vi "TCPSYN.vi"(5 "vi reference":refnum<vi>, 6 "Front Panel Window:Open":bool, 7 "error in vi ref":errorcluster, 8 "error in TCP":errorcluster, 9 "input Controls":cluster{"name":string, "type desc":i16[]}[](array[cluster]), 10 "input Indicators":cluster{"name":string, "type desc":i16[]}[](array[cluster]), 11 "connection ID in":refnum<k5>) -> (0 "error TCP out":errorcluster, 1 "error out":errorcluster, 2 "vi reference":refnum<vi>, 3 "connection ID out":refnum<k5>)   [LabVIEW 2010]
panel:
  out "error out 2":errorcluster
types:
  T1 = enum32{"Bad", "Idle", "Run top level", "Running"}
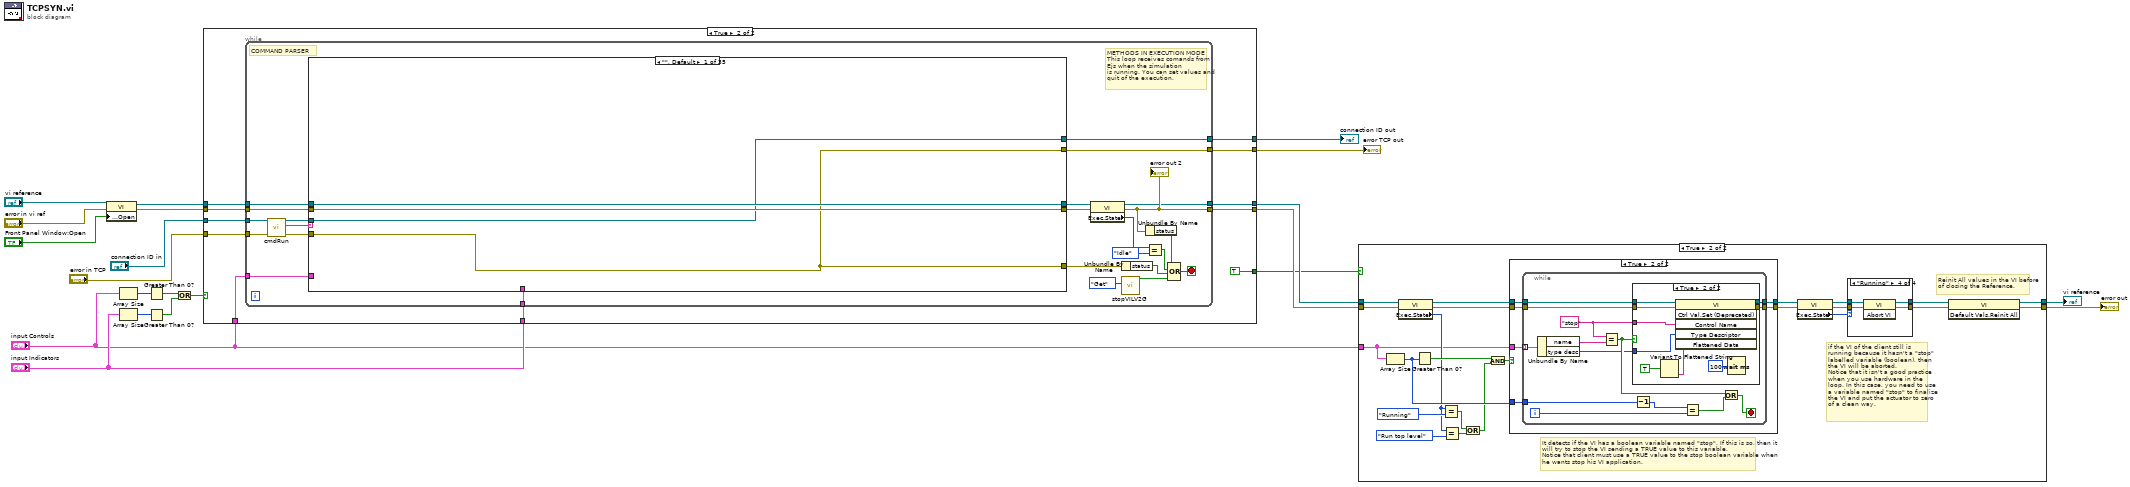
[diagram p0: block diagram]
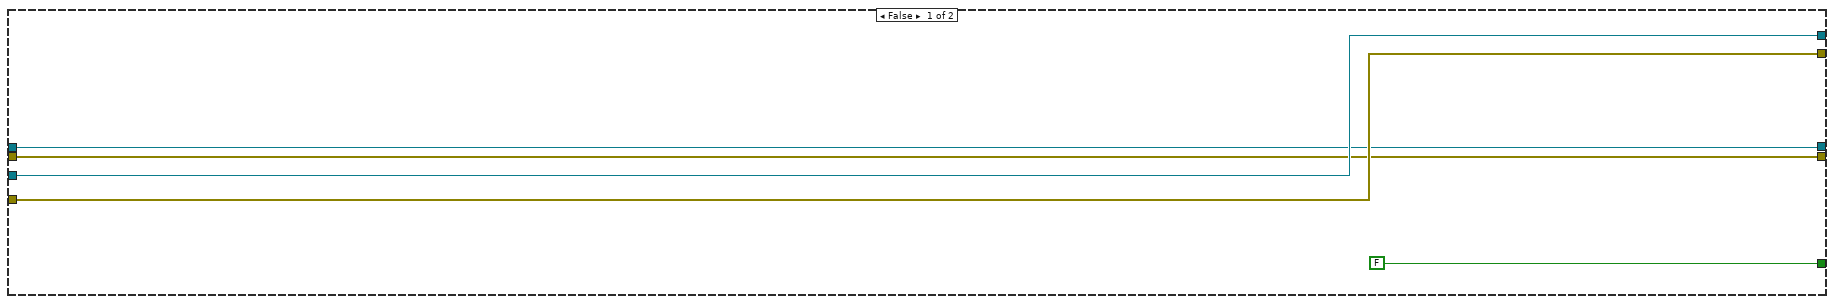
[diagram p8: hidden frame]
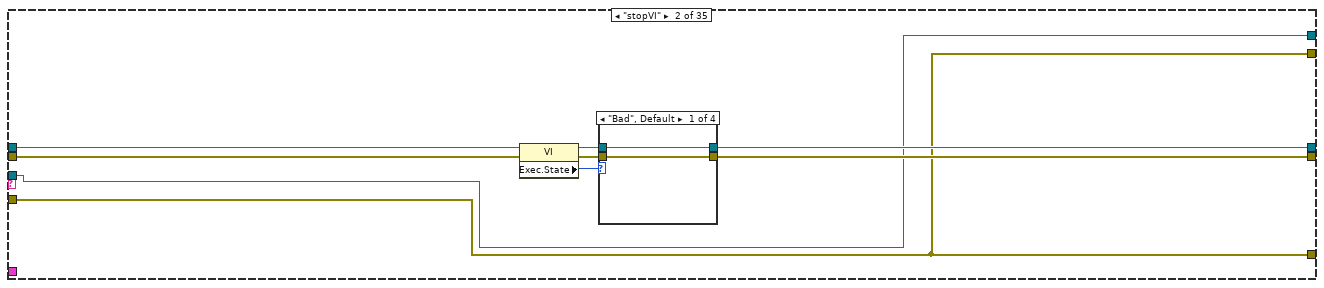
[diagram p9: hidden frame]
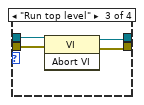
[diagram p11: hidden frame]
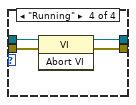
[diagram p12: hidden frame]
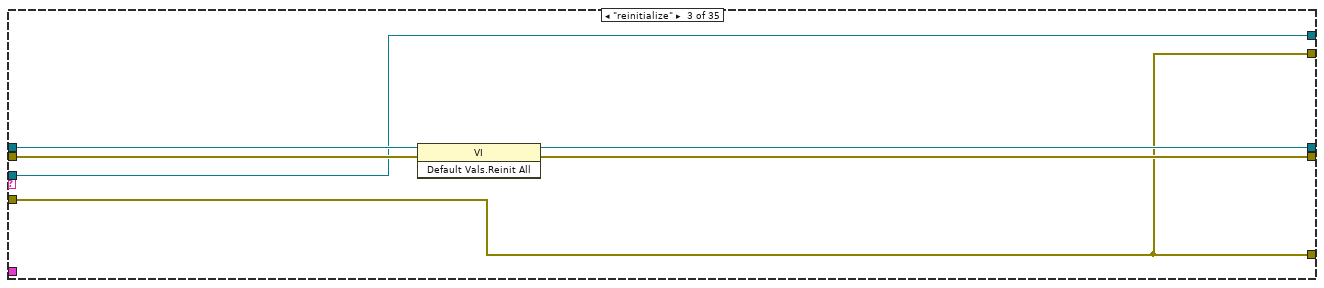
[diagram p13: hidden frame]
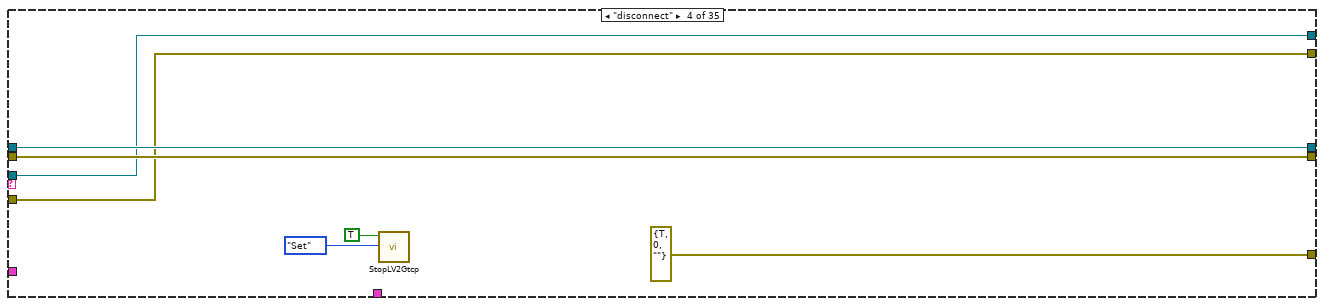
[diagram p14: hidden frame]
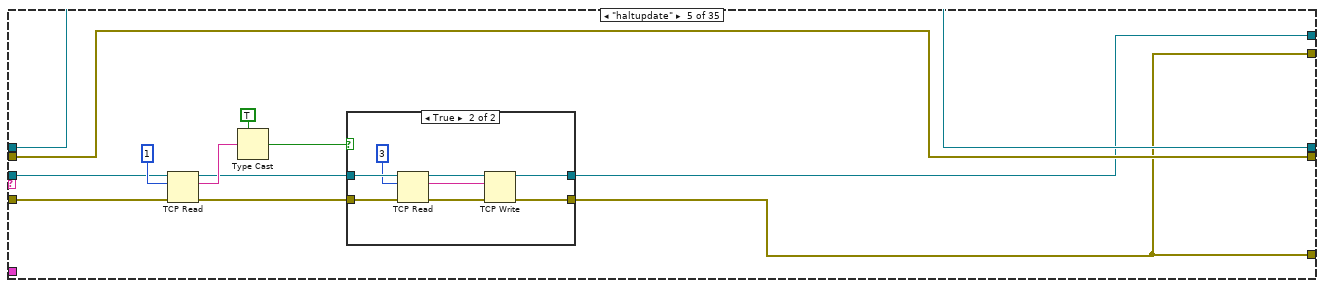
[diagram p15: hidden frame]
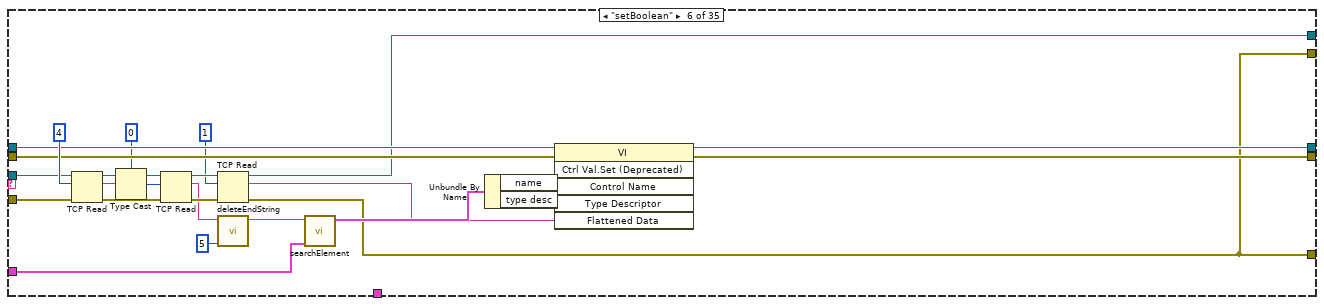
[diagram p17: hidden frame]
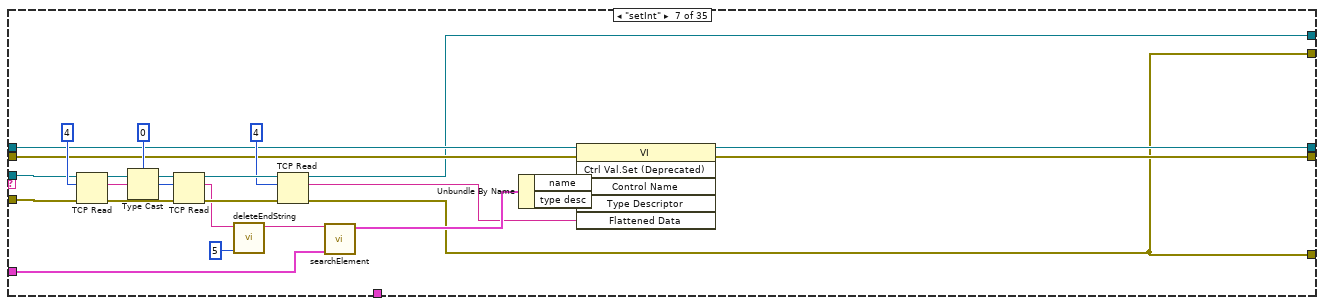
[diagram p18: hidden frame]
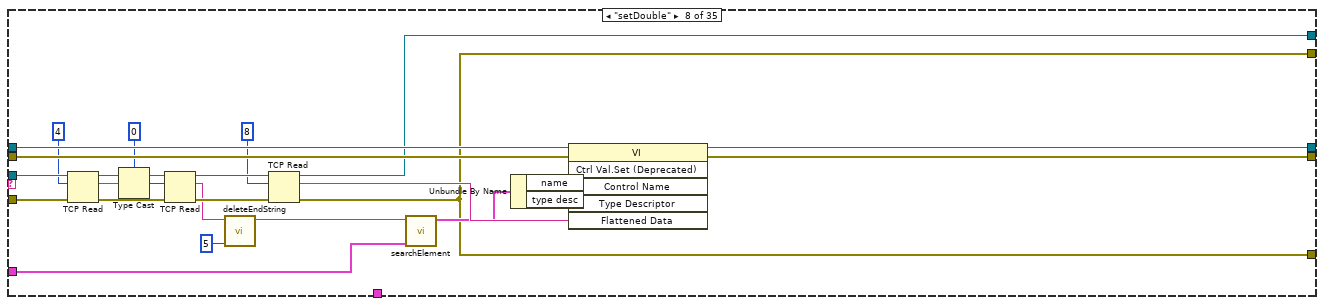
[diagram p19: hidden frame]
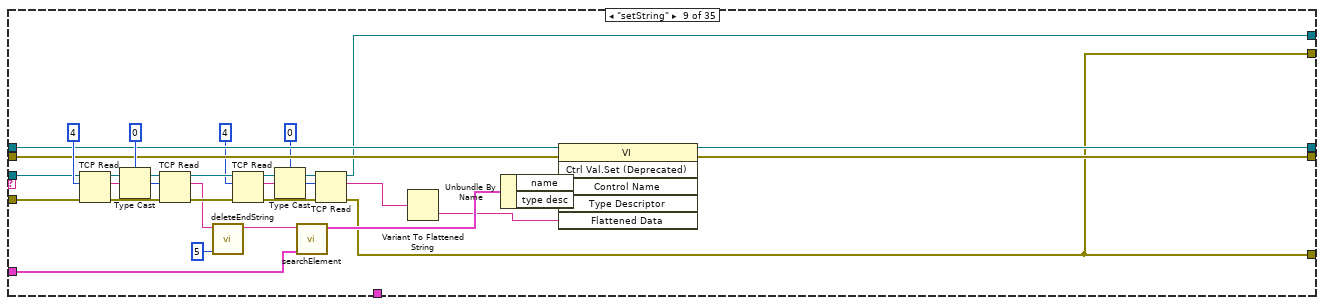
[diagram p20: hidden frame]
diagram:
  n1 = property on="Property Node" class="VI"(reference="vi reference", error in="error in vi ref", "Front Panel.Open"="Front Panel Window:Open") -> (reference out=w15:refnum<vi>, error out=w16:errorcluster)
  n2 = Array Size(array="input Controls") -> (size(s)=w14:i32)
  n3 = Array Size(array="input Indicators") -> (size(s)=w12:i32)
  n4 = Greater Than 0?(x=w14) -> (x > 0?=w13:bool)
  n5 = Greater Than 0?(x=w12) -> (x > 0?=w11:bool)
  n6 = Or(x=w13, y=w11) -> (x .or. y?=w9:bool)
  n7 = case shown="True" w9 {
    tunnel: "connection ID in" -> [w25 w37]
    tunnel: "error in TCP" -> [w24 w36]
    tunnel: "input Controls" -> [_ w35]
    tunnel: "input Indicators" -> [_ w34]
    tunnel: w15 -> [w23 w33]
    tunnel: w16 -> [w22 w32]
    tunnel: [FALSE TRUE] -> w2
    tunnel: [w22 w30] -> w4
    tunnel: [w23 w29] -> w3
    tunnel: [w25 w28] -> w8
    tunnel: [w24 w27] -> w7
    frame False {
    }
    frame True {
      n8 = while {
        tunnel: w37 -> [w58]
        tunnel: w36 -> [w57]
        tunnel: w33 -> [w61]
        tunnel: w32 -> [w60]
        tunnel: w35 -> [w52]
        tunnel: w34 -> [w43]
        tunnel: [w41] -> w30
        tunnel: [w40] -> w29
        tunnel: [w39] -> w28
        tunnel: [w38] -> w27
        stop <- w42 stop-if-true
        # "METHODS IN EXECUTION MODE\nThis loop receives comands from Ejs when the simulation\nis running. You can set values and quit of the execution."
        # "COMMAND PARSER"
        n9 = call "cmdRun.vi"("error in (no error)"=w57, "connection ID"=w58) -> ("error out"=w54:errorcluster, "Command"=w56:string, "connection ID out"=w55:refnum<k5>)  [unwired: 7 out]
        n10 = case shown="\"\", Default" w56 {
          tunnel: w61 -> [w64 w71 w92 w96 w103 w142 w152 w196 w216 w236 w256 w292 w341 _ w409 w441 w482 w530 w564 w620 w657 w684 w707 w725 w753 w773 w796 w819 w842 w867 w888 w911 w934 w957 w978]
          tunnel: w60 -> [w65 w70 w91 w95 w102 w141 w149 w195 w215 w235 w255 w291 w340 _ w408 w440 w481 w531 w563 w619 w656 w683 w706 w726 w752 w772 w797 w820 w843 w868 w889 w912 w935 w958 w977]
          tunnel: [w65 w68 w89 w95 w102 w139 w151 w194 w211 w232 w259 w293 w339 w363 w403 w442 w484 w528 w565 w615 w658 w681 w704 w728 w747 w770 w795 w818 w841 w862 w887 w910 w933 w956 w980] -> w48
          tunnel: w55 -> [w63 w67 w87 w93 w104 w138 w159 w192 w214 w231 w262 w296 w349 w367 w406 w445 w487 w545 w568 w618 w661 w679 w703 w730 w751 w774 w799 w821 w845 w866 w890 w914 w936 w959 w983]
          tunnel: w54 -> [w62 w66 w88 w94 w105 w137 w160 w193 w213 w230 w261 w295 w348 w366 w407 w444 w486 w544 w567 w617 w660 w678 w702 w729 w750 w775 w798 w822 w844 w865 w891 w913 w937 w960 w982]
          tunnel: [w62 w66 w88 errorcluster {"status"=TRUE, "code"=0, "source"=""} ("error out") w100 w123 w147 w172 w197 w228 w254 w290 w326 w361 w402 w437 w478 w519 w560 w612 w653 w676 w699 w722 w745 w768 w791 w814 w837 w860 w883 w906 w929 w952 w975] -> w53
          tunnel: w52 -> [_ _ _ _ _ w140 w154 w182 w212 w234 w258 w297 w344 w365 w405 w439 w483 w543 w562 w614 _ _ _ _ _ _ _ _ _ _ _ _ _ _ _]
          tunnel: [w64 w69 w90 w96 w103 w124 w150 w174 w199 w233 w260 w294 w327 w364 w404 w443 w485 w521 w566 w616 w659 w682 w705 w727 w748 w771 w794 w817 w840 w863 w886 w909 w932 w955 w979] -> w49
          tunnel: w43 -> [_ _ _ _ _ _ _ _ _ _ _ _ _ _ _ _ _ _ _ _ w655 w680 w701 w724 w749 w776 w793 w816 w839 w864 w885 w908 w931 w954 w981]
          tunnel: [w63 w67 w87 w93 w101 w122 w148 w173 w198 w229 w253 w289 w325 w362 w401 w438 w479 w520 w561 w613 w654 w677 w700 w723 w746 w769 w792 w815 w838 w861 w884 w907 w930 w953 w976] -> w39
          tunnel: [w62 w66 w88 w94 w100 w123 w147 w172 w197 w228 w254 w290 w326 w361 w402 w437 w478 w519 w560 w612 w653 w676 w699 w722 w745 w768 w791 w814 w837 w860 w883 w906 w929 w952 w975] -> w38
          frame "", Default {
          }
          frame "stopVI" {
            n11 = property class="VI"(reference=w71, error in=w70) -> (reference out=w73:refnum<vi>, error out=w72:errorcluster, "Exec.State"=w74:T1)
            n12 = case shown="\"Bad\", Default" w74 {
              tunnel: w73 -> [w76 w78 w82 w86]
              tunnel: w72 -> [w75 w77 w81 w85]
              tunnel: [w76 w78 w80 w84] -> w69
              tunnel: [w75 w77 w79 w83] -> w68
              frame "Bad", Default {
              }
              frame "Idle" {
              }
              frame "Run top level" {
                n13 = invoke class="VI" method="Abort VI"(reference=w82, error in=w81) -> (reference out=w80:refnum<vi>, error out=w79:errorcluster)  [unwired: 1 in, 1 out]
              }
              frame "Running" {
                n14 = invoke class="VI" method="Abort VI"(reference=w86, error in=w85) -> (reference out=w84:refnum<vi>, error out=w83:errorcluster)  [unwired: 1 in, 1 out]
              }
            }
          }
          frame "reinitialize" {
            n15 = invoke class="VI" method="Default Vals.Reinit All"(reference=w92, error in=w91) -> (reference out=w90:refnum<vi>, error out=w89:errorcluster)  [unwired: 1 in, 1 out]
          }
          frame "disconnect" {
            n16 = call "StopLV2Gtcp.vi"("Mode"=enum16{"Init", "Get", "Set"}."Set", "Stop IN"=TRUE) -> ()  [unwired: 10 out]
          }
          frame "haltupdate" {
            n17 = TCP Read(connection ID=w104, bytes to read=1, error in (no error)=w105) -> (connection ID out=w107:refnum<k5>, data out=w110:string, error out=w106:errorcluster)  [unwired: 2 out]
            n18 = Type Cast(type=TRUE, x=w110) -> (*(type *) &x=w108:bool)
            n19 = case shown="True" w108 {
              tunnel: w107 -> [w112 w121]
              tunnel: w106 -> [w113 w120]
              tunnel: [w113 w115] -> w100
              tunnel: [w112 w114] -> w101
              frame False {
              }
              frame True {
                n20 = TCP Read(connection ID=w121, bytes to read=3, error in (no error)=w120) -> (connection ID out=w119:refnum<k5>, data out=w117:string, error out=w118:errorcluster)  [unwired: 2 out]
                n21 = TCP Write(connection ID=w119, data in=w117, error in (no error)=w118) -> (connection ID out=w114:refnum<k5>, error out=w115:errorcluster)  [unwired: 2 out]
              }
            }
          }
          frame "setBoolean" {
            n22 = TCP Read(connection ID=w138, bytes to read=4, error in (no error)=w137) -> (connection ID out=w133:refnum<k5>, data out=w136:string, error out=w132:errorcluster)  [unwired: 2 out]
            n23 = Type Cast(type=0, x=w136) -> (*(type *) &x=w134:i32)
            n24 = TCP Read(connection ID=w133, bytes to read=w134, error in (no error)=w132) -> (connection ID out=w130:refnum<k5>, data out=w127:string, error out=w131:errorcluster)  [unwired: 2 out]
            n25 = TCP Read(connection ID=w130, bytes to read=1, error in (no error)=w131) -> (connection ID out=w122:refnum<k5>, data out=w128:string, error out=w123:errorcluster)  [unwired: 2 out]
            n26 = call "deleteEndString.vi"("chars to delete"=5, "string in"=w127) -> ("substring out"=w126:string)  [unwired: 9 out]
            n27 = call "searchElement.vi"("input"=w140, "name"=w126) -> ("output"=w145:cluster{"name":string, "type desc":i16[]})  [unwired: 9 out]
            n28 = Unbundle By Name(w145) -> ("name"=w144:string, "type desc"=w143:i16[])
            n29 = invoke class="VI" method="Ctrl Val.Set (Deprecated)"(reference=w142, error in=w141, "Control Name"=w144, "Type Descriptor"=w143, "Flattened Data"=w128) -> (reference out=w124:refnum<vi>, error out=w139:errorcluster)  [unwired: 1 in, 4 out]
          }
          frame "setInt" {
            n30 = TCP Read(connection ID=w159, bytes to read=4, error in (no error)=w160) -> (connection ID out=w168:refnum<k5>, data out=w167:string, error out=w170:errorcluster)  [unwired: 2 out]
            n31 = Type Cast(type=0, x=w167) -> (*(type *) &x=w166:i32)
            n32 = TCP Read(connection ID=w168, bytes to read=w166, error in (no error)=w170) -> (connection ID out=w165:refnum<k5>, data out=w161:string, error out=w164:errorcluster)  [unwired: 2 out]
            n33 = call "deleteEndString.vi"("chars to delete"=5 ("y"), "string in"=w161) -> ("substring out"=w153:string)  [unwired: 9 out]
            n34 = TCP Read(connection ID=w165, bytes to read=4, error in (no error)=w164) -> (connection ID out=w148:refnum<k5>, data out=w155:string, error out=w147:errorcluster)  [unwired: 2 out]
            n35 = call "searchElement.vi"("input"=w154, "name"=w153) -> ("output"=w158:cluster{"name":string, "type desc":i16[]})  [unwired: 9 out]
            n36 = Unbundle By Name(w158) -> ("name"=w157:string, "type desc"=w156:i16[])
            n37 = invoke class="VI" method="Ctrl Val.Set (Deprecated)"(reference=w152, error in=w149, "Control Name"=w157, "Type Descriptor"=w156, "Flattened Data"=w155) -> (reference out=w150:refnum<vi>, error out=w151:errorcluster)  [unwired: 1 in, 4 out]
          }
          frame "setDouble" {
            n38 = TCP Read(connection ID=w192, bytes to read=4, error in (no error)=w193) -> (connection ID out=w188:refnum<k5>, data out=w187:string, error out=w190:errorcluster)  [unwired: 2 out]
            n39 = Type Cast(type=0, x=w187) -> (*(type *) &x=w186:i32)
            n40 = TCP Read(connection ID=w188, bytes to read=w186, error in (no error)=w190) -> (connection ID out=w185:refnum<k5>, data out=w176:string, error out=w184:errorcluster)  [unwired: 2 out]
            n41 = call "deleteEndString.vi"("chars to delete"=5 ("y"), "string in"=w176) -> ("substring out"=w175:string)  [unwired: 9 out]
            n42 = TCP Read(connection ID=w185, bytes to read=8, error in (no error)=w184) -> (connection ID out=w173:refnum<k5>, data out=w183:string, error out=w172:errorcluster)  [unwired: 2 out]
            n43 = call "searchElement.vi"("input"=w182, "name"=w175) -> ("output"=w181:cluster{"name":string, "type desc":i16[]})  [unwired: 9 out]
            n44 = Unbundle By Name(w181) -> ("name"=w180:string, "type desc"=w179:i16[])
            n45 = invoke class="VI" method="Ctrl Val.Set (Deprecated)"(reference=w196, error in=w195, "Control Name"=w180, "Type Descriptor"=w179, "Flattened Data"=w183) -> (reference out=w174:refnum<vi>, error out=w194:errorcluster)  [unwired: 1 in, 4 out]
          }
          frame "setString" {
            n46 = TCP Read(connection ID=w214, bytes to read=4, error in (no error)=w213) -> (connection ID out=w224:refnum<k5>, data out=w223:string, error out=w226:errorcluster)  [unwired: 2 out]
            n47 = Type Cast(type=0, x=w223) -> (*(type *) &x=w222:i32)
            n48 = TCP Read(connection ID=w224, bytes to read=w222, error in (no error)=w226) -> (connection ID out=w221:refnum<k5>, data out=w204:string, error out=w220:errorcluster)  [unwired: 2 out]
            n49 = call "deleteEndString.vi"("chars to delete"=5, "string in"=w204) -> ("substring out"=w202:string)  [unwired: 9 out]
            n50 = TCP Read(connection ID=w221, bytes to read=4, error in (no error)=w220) -> (connection ID out=w208:refnum<k5>, data out=w206:string, error out=w209:errorcluster)  [unwired: 2 out]
            n51 = Type Cast(type=0, x=w206) -> (*(type *) &x=w205:i32)
            n52 = call "searchElement.vi"("input"=w212, "name"=w202) -> ("output"=w219:cluster{"name":string, "type desc":i16[]})  [unwired: 9 out]
            n53 = TCP Read(connection ID=w208, bytes to read=w205, error in (no error)=w209) -> (connection ID out=w198:refnum<k5>, data out=w201:string, error out=w197:errorcluster)  [unwired: 2 out]
            n54 = Variant To Flattened String(Variant=w201) -> (data string=w200:string)  [unwired: 1 out]
            n55 = Unbundle By Name(w219) -> ("name"=w218:string, "type desc"=w217:i16[])
            n56 = invoke class="VI" method="Ctrl Val.Set (Deprecated)"(reference=w216, error in=w215, "Control Name"=w218, "Type Descriptor"=w217, "Flattened Data"=w200) -> (reference out=w199:refnum<vi>, error out=w211:errorcluster)  [unwired: 1 in, 4 out]
          }
          frame "setFloat" {
            n57 = TCP Read(connection ID=w231, bytes to read=4, error in (no error)=w230) -> (connection ID out=w249:refnum<k5>, data out=w248:string, error out=w251:errorcluster)  [unwired: 2 out]
            n58 = Type Cast(type=0, x=w248) -> (*(type *) &x=w247:i32)
            n59 = TCP Read(connection ID=w249, bytes to read=w247, error in (no error)=w251) -> (connection ID out=w246:refnum<k5>, data out=w238:string, error out=w245:errorcluster)  [unwired: 2 out]
            n60 = call "deleteEndString.vi"("chars to delete"=5 ("y"), "string in"=w238) -> ("substring out"=w237:string)  [unwired: 9 out]
            n61 = TCP Read(connection ID=w246, bytes to read=4, error in (no error)=w245) -> (connection ID out=w229:refnum<k5>, data out=w244:string, error out=w228:errorcluster)  [unwired: 2 out]
            n62 = call "searchElement.vi"("input"=w234, "name"=w237) -> ("output"=w243:cluster{"name":string, "type desc":i16[]})  [unwired: 9 out]
            n63 = Unbundle By Name(w243) -> ("name"=w242:string, "type desc"=w241:i16[])
            n64 = invoke class="VI" method="Ctrl Val.Set (Deprecated)"(reference=w236, error in=w235, "Control Name"=w242, "Type Descriptor"=w241, "Flattened Data"=w244) -> (reference out=w233:refnum<vi>, error out=w232:errorcluster)  [unwired: 1 in, 4 out]
          }
          frame "setBooleanArray" {
            n65 = TCP Read(connection ID=w262, bytes to read=4, error in (no error)=w261) -> (connection ID out=w286:refnum<k5>, data out=w285:string, error out=w288:errorcluster)  [unwired: 2 out]
            n66 = Type Cast(type=0, x=w285) -> (*(type *) &x=w284:i32)
            n67 = TCP Read(connection ID=w286, bytes to read=w284, error in (no error)=w288) -> (connection ID out=w283:refnum<k5>, data out=w275:string, error out=w282:errorcluster)  [unwired: 2 out]
            n68 = call "deleteEndString.vi"("chars to delete"=5 ("y"), "string in"=w275) -> ("substring out"=w276:string)  [unwired: 9 out]
            n69 = TCP Read(connection ID=w283, bytes to read=4, error in (no error)=w282) -> (connection ID out=w280:refnum<k5>, data out=w278:string, error out=w281:errorcluster)  [unwired: 2 out]
            n70 = Type Cast(type=0, x=w278) -> (*(type *) &x=w269:i32)
            n71 = Multiply(x=1, y=w269) -> (x*y=w271:i32)
            n72 = call "searchElement.vi"("input"=w258, "name"=w276) -> ("output"=w272:cluster{"name":string, "type desc":i16[]})  [unwired: 9 out]
            n73 = TCP Read(connection ID=w280, bytes to read=w271, error in (no error)=w281) -> (connection ID out=w253:refnum<k5>, data out=w267:string, error out=w254:errorcluster)  [unwired: 2 out]
            n74 = Unflatten From String(type=bool[] [], binary string=w267, data includes array or string size? (T)=FALSE) -> (value=w265:bool[])  [unwired: 1 in, 3 out]
            n75 = Variant To Flattened String(Variant=w265) -> (data string=w268:string)  [unwired: 1 out]
            n76 = Unbundle By Name(w272) -> ("name"=w274:string, "type desc"=w273:i16[])
            n77 = invoke class="VI" method="Ctrl Val.Set (Deprecated)"(reference=w256, error in=w255, "Control Name"=w274, "Type Descriptor"=w273, "Flattened Data"=w268) -> (reference out=w260:refnum<vi>, error out=w259:errorcluster)  [unwired: 1 in, 4 out]
          }
          frame "setIntArray" {
            n78 = TCP Read(connection ID=w296, bytes to read=4, error in (no error)=w295) -> (connection ID out=w322:refnum<k5>, data out=w321:string, error out=w324:errorcluster)  [unwired: 2 out]
            n79 = Type Cast(type=0, x=w321) -> (*(type *) &x=w320:i32)
            n80 = TCP Read(connection ID=w322, bytes to read=w320, error in (no error)=w324) -> (connection ID out=w319:refnum<k5>, data out=w311:string, error out=w318:errorcluster)  [unwired: 2 out]
            n81 = call "deleteEndString.vi"("chars to delete"=5 ("y"), "string in"=w311) -> ("substring out"=w312:string)  [unwired: 9 out]
            n82 = TCP Read(connection ID=w319, bytes to read=4, error in (no error)=w318) -> (connection ID out=w316:refnum<k5>, data out=w314:string, error out=w317:errorcluster)  [unwired: 2 out]
            n83 = Type Cast(type=0, x=w314) -> (*(type *) &x=w305:i32)
            n84 = Multiply(x=4, y=w305) -> (x*y=w307:i32)
            n85 = call "searchElement.vi"("input"=w297, "name"=w312) -> ("output"=w308:cluster{"name":string, "type desc":i16[]})  [unwired: 9 out]
            n86 = TCP Read(connection ID=w316, bytes to read=w307, error in (no error)=w317) -> (connection ID out=w289:refnum<k5>, data out=w303:string, error out=w290:errorcluster)  [unwired: 2 out]
            n87 = Unflatten From String(type=i32[] [], binary string=w303, data includes array or string size? (T)=FALSE) -> (value=w300:i32[])  [unwired: 1 in, 3 out]
            n88 = Variant To Flattened String(Variant=w300) -> (data string=w304:string)  [unwired: 1 out]
            n89 = Unbundle By Name(w308) -> ("name"=w310:string, "type desc"=w309:i16[])
            n90 = invoke class="VI" method="Ctrl Val.Set (Deprecated)"(reference=w292, error in=w291, "Control Name"=w310, "Type Descriptor"=w309, "Flattened Data"=w304) -> (reference out=w294:refnum<vi>, error out=w293:errorcluster)  [unwired: 1 in, 4 out]
          }
          frame "setDoubleArray" {
            n91 = TCP Read(connection ID=w349, bytes to read=4, error in (no error)=w348) -> (connection ID out=w358:refnum<k5>, data out=w357:string, error out=w360:errorcluster)  [unwired: 2 out]
            n92 = Type Cast(type=0, x=w357) -> (*(type *) &x=w356:i32)
            n93 = TCP Read(connection ID=w358, bytes to read=w356, error in (no error)=w360) -> (connection ID out=w355:refnum<k5>, data out=w345:string, error out=w354:errorcluster)  [unwired: 2 out]
            n94 = call "deleteEndString.vi"("chars to delete"=5 ("y"), "string in"=w345) -> ("substring out"=w346:string)  [unwired: 9 out]
            n95 = TCP Read(connection ID=w355, bytes to read=4, error in (no error)=w354) -> (connection ID out=w352:refnum<k5>, data out=w350:string, error out=w353:errorcluster)  [unwired: 2 out]
            n96 = Type Cast(type=0, x=w350) -> (*(type *) &x=w335:i32)
            n97 = Multiply(x=8, y=w335) -> (x*y=w337:i32)
            n98 = call "searchElement.vi"("input"=w344, "name"=w346) -> ("output"=w338:cluster{"name":string, "type desc":i16[]})  [unwired: 9 out]
            n99 = TCP Read(connection ID=w352, bytes to read=w337, error in (no error)=w353) -> (connection ID out=w325:refnum<k5>, data out=w333:string, error out=w326:errorcluster)  [unwired: 2 out]
            n100 = Unflatten From String(type=dbl[] [], binary string=w333, data includes array or string size? (T)=FALSE) -> (value=w330:dbl[])  [unwired: 1 in, 3 out]
            n101 = Variant To Flattened String(Variant=w330) -> (data string=w334:string)  [unwired: 1 out]
            n102 = Unbundle By Name(w338) -> ("name"=w343:string, "type desc"=w342:i16[])
            n103 = invoke class="VI" method="Ctrl Val.Set (Deprecated)"(reference=w341, error in=w340, "Control Name"=w343, "Type Descriptor"=w342, "Flattened Data"=w334) -> (reference out=w327:refnum<vi>, error out=w339:errorcluster)  [unwired: 1 in, 4 out]
          }
          frame "setStringArray" {
            n104 = TCP Read(connection ID=w367, bytes to read=4, error in (no error)=w366) -> (connection ID out=w387:refnum<k5>, data out=w386:string, error out=w389:errorcluster)  [unwired: 2 out]
            n105 = Type Cast(type=0, x=w386) -> (*(type *) &x=w385:i32)
            n106 = TCP Read(connection ID=w387, bytes to read=w385, error in (no error)=w389) -> (connection ID out=w384:refnum<k5>, data out=w378:string, error out=w383:errorcluster)  [unwired: 2 out]
            n107 = TCP Read(connection ID=w384, bytes to read=4, error in (no error)=w383) -> (connection ID out=w370:refnum<k5>, data out=w381:string, error out=w369:errorcluster)  [unwired: 2 out]
            n108 = Type Cast(type=0, x=w381) -> (*(type *) &x=w371:i32)
            n109 = call "deleteEndString.vi"("chars to delete"=5 ("y"), "string in"=w378) -> ("substring out"=w379:string)  [unwired: 9 out]
            n110 = for {
              N: w371 -> [_]
              tunnel: w370 -> [w400]
              tunnel: w369 -> [w399]
              tunnel: [w392] -> w362
              tunnel: [w391] -> w361
              tunnel: [w390] -> w368 mode=indexing
              n111 = TCP Read(connection ID=w400, bytes to read=4, error in (no error)=w399) -> (connection ID out=w397:refnum<k5>, data out=w394:string, error out=w396:errorcluster)  [unwired: 2 out]
              n112 = Type Cast(type=0, x=w394) -> (*(type *) &x=w393:i32)
              n113 = TCP Read(connection ID=w397, bytes to read=w393, error in (no error)=w396) -> (connection ID out=w392:refnum<k5>, data out=w390:string, error out=w391:errorcluster)  [unwired: 2 out]
            }
            n114 = call "searchElement.vi"("input"=w365, "name"=w379) -> ("output"=w375:cluster{"name":string, "type desc":i16[]})  [unwired: 9 out]
            n115 = Variant To Flattened String(Variant=w368) -> (data string=w374:string)  [unwired: 1 out]
            n116 = Unbundle By Name(w375) -> ("name"=w377:string, "type desc"=w376:i16[])
            n117 = invoke class="VI" method="Ctrl Val.Set (Deprecated)"("Control Name"=w377, "Type Descriptor"=w376, "Flattened Data"=w374) -> (reference out=w364:refnum<vi>, error out=w363:errorcluster)  [unwired: 3 in, 4 out]
          }
          frame "setFloatArray" {
            n118 = TCP Read(connection ID=w406, bytes to read=4, error in (no error)=w407) -> (connection ID out=w434:refnum<k5>, data out=w433:string, error out=w436:errorcluster)  [unwired: 2 out]
            n119 = Type Cast(type=0, x=w433) -> (*(type *) &x=w432:i32)
            n120 = TCP Read(connection ID=w434, bytes to read=w432, error in (no error)=w436) -> (connection ID out=w431:refnum<k5>, data out=w423:string, error out=w430:errorcluster)  [unwired: 2 out]
            n121 = call "deleteEndString.vi"("chars to delete"=5 ("y"), "string in"=w423) -> ("substring out"=w424:string)  [unwired: 9 out]
            n122 = TCP Read(connection ID=w431, bytes to read=4, error in (no error)=w430) -> (connection ID out=w428:refnum<k5>, data out=w426:string, error out=w429:errorcluster)  [unwired: 2 out]
            n123 = Type Cast(type=0, x=w426) -> (*(type *) &x=w417:i32)
            n124 = Multiply(x=4, y=w417) -> (x*y=w419:i32)
            n125 = call "searchElement.vi"("input"=w405, "name"=w424) -> ("output"=w420:cluster{"name":string, "type desc":i16[]})  [unwired: 9 out]
            n126 = TCP Read(connection ID=w428, bytes to read=w419, error in (no error)=w429) -> (connection ID out=w401:refnum<k5>, data out=w415:string, error out=w402:errorcluster)  [unwired: 2 out]
            n127 = Unflatten From String(type=sgl[] [], binary string=w415, data includes array or string size? (T)=FALSE) -> (value=w412:sgl[])  [unwired: 1 in, 3 out]
            n128 = Variant To Flattened String(Variant=w412) -> (data string=w416:string)  [unwired: 1 out]
            n129 = Unbundle By Name(w420) -> ("name"=w422:string, "type desc"=w421:i16[])
            n130 = invoke class="VI" method="Ctrl Val.Set (Deprecated)"(reference=w409, error in=w408, "Control Name"=w422, "Type Descriptor"=w421, "Flattened Data"=w416) -> (reference out=w404:refnum<vi>, error out=w403:errorcluster)  [unwired: 1 in, 4 out]
          }
          frame "setBooleanArray2D" {
            w464 = 4 ("bytes to read")
            n131 = TCP Read(connection ID=w445, bytes to read=4, error in (no error)=w444) -> (connection ID out=w474:refnum<k5>, data out=w473:string, error out=w476:errorcluster)  [unwired: 2 out]
            n132 = Type Cast(type=0, x=w473) -> (*(type *) &x=w472:i32)
            n133 = TCP Read(connection ID=w474, bytes to read=w472, error in (no error)=w476) -> (connection ID out=w471:refnum<k5>, data out=w465:string, error out=w470:errorcluster)  [unwired: 2 out]
            n134 = TCP Read(connection ID=w471, bytes to read=w464, error in (no error)=w470) -> (connection ID out=w468:refnum<k5>, data out=w463:string, error out=w469:errorcluster)  [unwired: 2 out]
            n135 = call "deleteEndString.vi"("chars to delete"=5 ("y"), "string in"=w465) -> ("substring out"=w466:string)  [unwired: 9 out]
            n136 = Type Cast(type=0, x=w463) -> (*(type *) &x=w457:i32)
            n137 = TCP Read(connection ID=w468, bytes to read=w464, error in (no error)=w469) -> (connection ID out=w460:refnum<k5>, data out=w461:string, error out=w459:errorcluster)  [unwired: 2 out]
            n138 = Type Cast(type=0, x=w461) -> (*(type *) &x=w458:i32)
            n139 = call "searchElement.vi"("input"=w439, "name"=w466) -> ("output"=w453:cluster{"name":string, "type desc":i16[]})  [unwired: 9 out]
            n140 = Compound Arithmetic op=MULTIPLY(w457, w458, 1 ("value")) -> (w456:i32)
            n141 = TCP Read(connection ID=w460, bytes to read=w456, error in (no error)=w459) -> (connection ID out=w438:refnum<k5>, data out=w451:string, error out=w437:errorcluster)  [unwired: 2 out]
            n142 = Unflatten From String(type=bool[][] [], binary string=w451, data includes array or string size? (T)=FALSE) -> (value=w450:bool[][])  [unwired: 1 in, 3 out]
            n143 = Variant To Flattened String(Variant=w450) -> (data string=w449:string)  [unwired: 1 out]
            n144 = Unbundle By Name(w453) -> ("name"=w455:string, "type desc"=w454:i16[])
            n145 = invoke class="VI" method="Ctrl Val.Set (Deprecated)"(reference=w441, error in=w440, "Control Name"=w455, "Type Descriptor"=w454, "Flattened Data"=w449) -> (reference out=w443:refnum<vi>, error out=w442:errorcluster)  [unwired: 1 in, 4 out]
          }
          frame "setIntArray2D" {
            w505 = 4 ("bytes to read")
            n146 = TCP Read(connection ID=w487, bytes to read=4, error in (no error)=w486) -> (connection ID out=w515:refnum<k5>, data out=w514:string, error out=w517:errorcluster)  [unwired: 2 out]
            n147 = Type Cast(type=0, x=w514) -> (*(type *) &x=w513:i32)
            n148 = TCP Read(connection ID=w515, bytes to read=w513, error in (no error)=w517) -> (connection ID out=w512:refnum<k5>, data out=w506:string, error out=w511:errorcluster)  [unwired: 2 out]
            n149 = TCP Read(connection ID=w512, bytes to read=w505, error in (no error)=w511) -> (connection ID out=w509:refnum<k5>, data out=w504:string, error out=w510:errorcluster)  [unwired: 2 out]
            n150 = Type Cast(type=0, x=w504) -> (*(type *) &x=w498:i32)
            n151 = call "deleteEndString.vi"("chars to delete"=5 ("y"), "string in"=w506) -> ("substring out"=w507:string)  [unwired: 9 out]
            n152 = TCP Read(connection ID=w509, bytes to read=w505, error in (no error)=w510) -> (connection ID out=w501:refnum<k5>, data out=w502:string, error out=w500:errorcluster)  [unwired: 2 out]
            n153 = Type Cast(type=0, x=w502) -> (*(type *) &x=w499:i32)
            n154 = call "searchElement.vi"("input"=w483, "name"=w507) -> ("output"=w494:cluster{"name":string, "type desc":i16[]})  [unwired: 9 out]
            n155 = Compound Arithmetic op=MULTIPLY(w498, w499, 4 ("value")) -> (w497:i32)
            n156 = TCP Read(connection ID=w501, bytes to read=w497, error in (no error)=w500) -> (connection ID out=w479:refnum<k5>, data out=w492:string, error out=w478:errorcluster)  [unwired: 2 out]
            n157 = Unflatten From String(type=i32[][] [], binary string=w492, data includes array or string size? (T)=FALSE) -> (value=w491:i32[][])  [unwired: 1 in, 3 out]
            n158 = Variant To Flattened String(Variant=w491) -> (data string=w490:string)  [unwired: 1 out]
            n159 = Unbundle By Name(w494) -> ("name"=w496:string, "type desc"=w495:i16[])
            n160 = invoke class="VI" method="Ctrl Val.Set (Deprecated)"(reference=w482, error in=w481, "Control Name"=w496, "Type Descriptor"=w495, "Flattened Data"=w490) -> (reference out=w485:refnum<vi>, error out=w484:errorcluster)  [unwired: 1 in, 4 out]
          }
          frame "setDoubleArray2D" {
            w542 = 4 ("bytes to read")
            n161 = TCP Read(connection ID=w545, bytes to read=4, error in (no error)=w544) -> (connection ID out=w556:refnum<k5>, data out=w555:string, error out=w558:errorcluster)  [unwired: 2 out]
            n162 = Type Cast(type=0, x=w555) -> (*(type *) &x=w554:i32)
            n163 = TCP Read(connection ID=w556, bytes to read=w554, error in (no error)=w558) -> (connection ID out=w553:refnum<k5>, data out=w546:string, error out=w552:errorcluster)  [unwired: 2 out]
            n164 = call "deleteEndString.vi"("chars to delete"=5 ("y"), "string in"=w546) -> ("substring out"=w547:string)  [unwired: 9 out]
            n165 = TCP Read(connection ID=w553, bytes to read=w542, error in (no error)=w552) -> (connection ID out=w550:refnum<k5>, data out=w541:string, error out=w551:errorcluster)  [unwired: 2 out]
            n166 = Type Cast(type=0, x=w541) -> (*(type *) &x=w535:i32)
            n167 = TCP Read(connection ID=w550, bytes to read=w542, error in (no error)=w551) -> (connection ID out=w538:refnum<k5>, data out=w539:string, error out=w537:errorcluster)  [unwired: 2 out]
            n168 = call "searchElement.vi"("input"=w543, "name"=w547) -> ("output"=w529:cluster{"name":string, "type desc":i16[]})  [unwired: 9 out]
            n169 = Type Cast(type=0, x=w539) -> (*(type *) &x=w536:i32)
            n170 = Compound Arithmetic op=MULTIPLY(w535, w536, 8 ("value")) -> (w534:i32)
            n171 = TCP Read(connection ID=w538, bytes to read=w534, error in (no error)=w537) -> (connection ID out=w520:refnum<k5>, data out=w526:string, error out=w519:errorcluster)  [unwired: 2 out]
            n172 = Unflatten From String(type=dbl[][] [], binary string=w526, data includes array or string size? (T)=FALSE) -> (value=w524:dbl[][])  [unwired: 1 in, 3 out]
            n173 = Unbundle By Name(w529) -> ("name"=w533:string, "type desc"=w532:i16[])
            n174 = Variant To Flattened String(Variant=w524) -> (data string=w523:string)  [unwired: 1 out]
            n175 = invoke class="VI" method="Ctrl Val.Set (Deprecated)"(reference=w530, error in=w531, "Control Name"=w533, "Type Descriptor"=w532, "Flattened Data"=w523) -> (reference out=w521:refnum<vi>, error out=w528:errorcluster)  [unwired: 1 in, 4 out]
          }
          frame "setStringArray2D" {
            w582 = 4 ("bytes to read")
            n176 = TCP Read(connection ID=w568, bytes to read=4, error in (no error)=w567) -> (connection ID out=w592:refnum<k5>, data out=w591:string, error out=w594:errorcluster)  [unwired: 2 out]
            n177 = Type Cast(type=0, x=w591) -> (*(type *) &x=w590:i32)
            n178 = TCP Read(connection ID=w592, bytes to read=w590, error in (no error)=w594) -> (connection ID out=w589:refnum<k5>, data out=w583:string, error out=w588:errorcluster)  [unwired: 2 out]
            n179 = TCP Read(connection ID=w589, bytes to read=w582, error in (no error)=w588) -> (connection ID out=w586:refnum<k5>, data out=w581:string, error out=w587:errorcluster)  [unwired: 2 out]
            n180 = call "deleteEndString.vi"("chars to delete"=5 ("y"), "string in"=w583) -> ("substring out"=w584:string)  [unwired: 9 out]
            n181 = Type Cast(type=0, x=w581) -> (*(type *) &x=w573:i32)
            n182 = TCP Read(connection ID=w586, bytes to read=w582, error in (no error)=w587) -> (connection ID out=w571:refnum<k5>, data out=w579:string, error out=w570:errorcluster)  [unwired: 2 out]
            n183 = call "searchElement.vi"("input"=w562, "name"=w584) -> ("output"=w576:cluster{"name":string, "type desc":i16[]})  [unwired: 9 out]
            n184 = Type Cast(type=0, x=w579) -> (*(type *) &x=w572:i32)
            n185 = for {
              N: w573 -> [_]
              tunnel: w572 -> [w601]
              tunnel: w571 -> [w600]
              tunnel: w570 -> [w599]
              tunnel: [w598] -> w561
              tunnel: [w597] -> w560
              tunnel: [w596] -> w569 mode=indexing
              n186 = for {
                N: w601 -> [_]
                tunnel: w600 -> [w611]
                tunnel: w599 -> [w610]
                tunnel: [w607] -> w598
                tunnel: [w606] -> w597
                tunnel: [w602] -> w596 mode=indexing
                n187 = TCP Read(connection ID=w611, error in (no error)=w610) -> (connection ID out=w609:refnum<k5>, data out=w604:string, error out=w608:errorcluster)  [unwired: 3 out]
                n188 = Type Cast(type=0, x=w604) -> (*(type *) &x=w603:i32)
                n189 = TCP Read(connection ID=w609, bytes to read=w603, error in (no error)=w608) -> (connection ID out=w607:refnum<k5>, data out=w602:string, error out=w606:errorcluster)  [unwired: 2 out]
              }
            }
            n190 = Variant To Flattened String(Variant=w569) -> (data string=w575:string)  [unwired: 1 out]
            n191 = Unbundle By Name(w576) -> ("name"=w578:string, "type desc"=w577:i16[])
            n192 = invoke class="VI" method="Ctrl Val.Set (Deprecated)"(reference=w564, error in=w563, "Control Name"=w578, "Type Descriptor"=w577, "Flattened Data"=w575) -> (reference out=w566:refnum<vi>, error out=w565:errorcluster)  [unwired: 1 in, 4 out]
          }
          frame "setFloatArray2D" {
            w638 = 4 ("bytes to read")
            n193 = TCP Read(connection ID=w618, bytes to read=4, error in (no error)=w617) -> (connection ID out=w649:refnum<k5>, data out=w648:string, error out=w651:errorcluster)  [unwired: 2 out]
            n194 = Type Cast(type=0, x=w648) -> (*(type *) &x=w647:i32)
            n195 = TCP Read(connection ID=w649, bytes to read=w647, error in (no error)=w651) -> (connection ID out=w646:refnum<k5>, data out=w639:string, error out=w645:errorcluster)  [unwired: 2 out]
            n196 = call "deleteEndString.vi"("chars to delete"=5 ("y"), "string in"=w639) -> ("substring out"=w640:string)  [unwired: 9 out]
            n197 = TCP Read(connection ID=w646, bytes to read=w638, error in (no error)=w645) -> (connection ID out=w643:refnum<k5>, data out=w637:string, error out=w644:errorcluster)  [unwired: 2 out]
            n198 = Type Cast(type=0, x=w637) -> (*(type *) &x=w631:i32)
            n199 = TCP Read(connection ID=w643, bytes to read=w638, error in (no error)=w644) -> (connection ID out=w634:refnum<k5>, data out=w635:string, error out=w633:errorcluster)  [unwired: 2 out]
            n200 = call "searchElement.vi"("input"=w614, "name"=w640) -> ("output"=w627:cluster{"name":string, "type desc":i16[]})  [unwired: 9 out]
            n201 = Type Cast(type=0, x=w635) -> (*(type *) &x=w632:i32)
            n202 = Compound Arithmetic op=MULTIPLY(w631, w632, 4 ("value")) -> (w630:i32)
            n203 = TCP Read(connection ID=w634, bytes to read=w630, error in (no error)=w633) -> (connection ID out=w613:refnum<k5>, data out=w625:string, error out=w612:errorcluster)  [unwired: 2 out]
            n204 = Unflatten From String(type=sgl[][] [], binary string=w625, data includes array or string size? (T)=FALSE) -> (value=w623:sgl[][])  [unwired: 1 in, 3 out]
            n205 = Unbundle By Name(w627) -> ("name"=w629:string, "type desc"=w628:i16[])
            n206 = Variant To Flattened String(Variant=w623) -> (data string=w622:string)  [unwired: 1 out]
            n207 = invoke class="VI" method="Ctrl Val.Set (Deprecated)"(reference=w620, error in=w619, "Control Name"=w629, "Type Descriptor"=w628, "Flattened Data"=w622) -> (reference out=w616:refnum<vi>, error out=w615:errorcluster)  [unwired: 1 in, 4 out]
          }
          frame "getBoolean" {
            n208 = TCP Read(connection ID=w661, bytes to read=4, error in (no error)=w660) -> (connection ID out=w669:refnum<k5>, data out=w672:string, error out=w668:errorcluster)  [unwired: 2 out]
            n209 = Type Cast(type=0, x=w672) -> (*(type *) &x=w670:i32)
            n210 = TCP Read(connection ID=w669, bytes to read=w670, error in (no error)=w668) -> (connection ID out=w664:refnum<k5>, data out=w667:string, error out=w663:errorcluster)  [unwired: 2 out]
            n211 = call "deleteEndString.vi"("chars to delete"=5, "string in"=w667) -> ("substring out"=w666:string)  [unwired: 9 out]
            n212 = call "searchElement.vi"("input"=w655, "name"=w666) -> ("output"=w674:cluster{"name":string, "type desc":i16[]})  [unwired: 9 out]
            n213 = Unbundle By Name(w674) -> ("name"=w673:string)
            n214 = invoke class="VI" method="Ctrl Val.Get (Deprecated)"(reference=w657, error in=w656, "Control Name"=w673) -> (reference out=w659:refnum<vi>, error out=w658:errorcluster, "Get Control Value"=w662:string)  [unwired: 2 in, 2 out]
            n215 = TCP Write(connection ID=w664, data in=w662, error in (no error)=w663) -> (connection ID out=w654:refnum<k5>, error out=w653:errorcluster)  [unwired: 2 out]
          }
          frame "getInt" {
            n216 = TCP Read(connection ID=w679, bytes to read=4, error in (no error)=w678) -> (connection ID out=w692:refnum<k5>, data out=w695:string, error out=w691:errorcluster)  [unwired: 2 out]
            n217 = Type Cast(type=0, x=w695) -> (*(type *) &x=w693:i32)
            n218 = TCP Read(connection ID=w692, bytes to read=w693, error in (no error)=w691) -> (connection ID out=w687:refnum<k5>, data out=w690:string, error out=w686:errorcluster)  [unwired: 2 out]
            n219 = call "deleteEndString.vi"("chars to delete"=5, "string in"=w690) -> ("substring out"=w689:string)  [unwired: 9 out]
            n220 = call "searchElement.vi"("input"=w680, "name"=w689) -> ("output"=w697:cluster{"name":string, "type desc":i16[]})  [unwired: 9 out]
            n221 = Unbundle By Name(w697) -> ("name"=w696:string)
            n222 = invoke class="VI" method="Ctrl Val.Get (Deprecated)"(reference=w684, error in=w683, "Control Name"=w696) -> (reference out=w682:refnum<vi>, error out=w681:errorcluster, "Get Control Value"=w685:string)  [unwired: 2 in, 2 out]
            n223 = TCP Write(connection ID=w687, data in=w685, error in (no error)=w686) -> (connection ID out=w677:refnum<k5>, error out=w676:errorcluster)  [unwired: 2 out]
          }
          frame "getDouble" {
            n224 = TCP Read(connection ID=w703, bytes to read=4, error in (no error)=w702) -> (connection ID out=w715:refnum<k5>, data out=w718:string, error out=w714:errorcluster)  [unwired: 2 out]
            n225 = Type Cast(type=0, x=w718) -> (*(type *) &x=w716:i32)
            n226 = TCP Read(connection ID=w715, bytes to read=w716, error in (no error)=w714) -> (connection ID out=w710:refnum<k5>, data out=w713:string, error out=w709:errorcluster)  [unwired: 2 out]
            n227 = call "deleteEndString.vi"("chars to delete"=5, "string in"=w713) -> ("substring out"=w712:string)  [unwired: 9 out]
            n228 = call "searchElement.vi"("input"=w701, "name"=w712) -> ("output"=w720:cluster{"name":string, "type desc":i16[]})  [unwired: 9 out]
            n229 = Unbundle By Name(w720) -> ("name"=w719:string)
            n230 = invoke class="VI" method="Ctrl Val.Get (Deprecated)"(reference=w707, error in=w706, "Control Name"=w719) -> (reference out=w705:refnum<vi>, error out=w704:errorcluster, "Get Control Value"=w708:string)  [unwired: 2 in, 2 out]
            n231 = TCP Write(connection ID=w710, data in=w708, error in (no error)=w709) -> (connection ID out=w700:refnum<k5>, error out=w699:errorcluster)  [unwired: 2 out]
          }
          frame "getString" {
            n232 = TCP Read(connection ID=w730, bytes to read=4, error in (no error)=w729) -> (connection ID out=w738:refnum<k5>, data out=w741:string, error out=w737:errorcluster)  [unwired: 2 out]
            n233 = Type Cast(type=0, x=w741) -> (*(type *) &x=w739:i32)
            n234 = TCP Read(connection ID=w738, bytes to read=w739, error in (no error)=w737) -> (connection ID out=w733:refnum<k5>, data out=w736:string, error out=w732:errorcluster)  [unwired: 2 out]
            n235 = call "deleteEndString.vi"("chars to delete"=5, "string in"=w736) -> ("substring out"=w735:string)  [unwired: 9 out]
            n236 = call "searchElement.vi"("input"=w724, "name"=w735) -> ("output"=w743:cluster{"name":string, "type desc":i16[]})  [unwired: 9 out]
            n237 = Unbundle By Name(w743) -> ("name"=w742:string)
            n238 = invoke class="VI" method="Ctrl Val.Get (Deprecated)"(reference=w725, error in=w726, "Control Name"=w742) -> (reference out=w727:refnum<vi>, error out=w728:errorcluster, "Get Control Value"=w731:string)  [unwired: 2 in, 2 out]
            n239 = TCP Write(connection ID=w733, data in=w731, error in (no error)=w732) -> (connection ID out=w723:refnum<k5>, error out=w722:errorcluster)  [unwired: 2 out]
          }
          frame "getFloat" {
            n240 = TCP Read(connection ID=w751, bytes to read=4, error in (no error)=w750) -> (connection ID out=w761:refnum<k5>, data out=w764:string, error out=w760:errorcluster)  [unwired: 2 out]
            n241 = Type Cast(type=0, x=w764) -> (*(type *) &x=w762:i32)
            n242 = TCP Read(connection ID=w761, bytes to read=w762, error in (no error)=w760) -> (connection ID out=w756:refnum<k5>, data out=w759:string, error out=w755:errorcluster)  [unwired: 2 out]
            n243 = call "deleteEndString.vi"("chars to delete"=5, "string in"=w759) -> ("substring out"=w758:string)  [unwired: 9 out]
            n244 = call "searchElement.vi"("input"=w749, "name"=w758) -> ("output"=w766:cluster{"name":string, "type desc":i16[]})  [unwired: 9 out]
            n245 = Unbundle By Name(w766) -> ("name"=w765:string)
            n246 = invoke class="VI" method="Ctrl Val.Get (Deprecated)"(reference=w753, error in=w752, "Control Name"=w765) -> (reference out=w748:refnum<vi>, error out=w747:errorcluster, "Get Control Value"=w754:string)  [unwired: 2 in, 2 out]
            n247 = TCP Write(connection ID=w756, data in=w754, error in (no error)=w755) -> (connection ID out=w746:refnum<k5>, error out=w745:errorcluster)  [unwired: 2 out]
          }
          frame "getBooleanArray" {
            n248 = TCP Read(connection ID=w774, bytes to read=4, error in (no error)=w775) -> (connection ID out=w784:refnum<k5>, data out=w787:string, error out=w783:errorcluster)  [unwired: 2 out]
            n249 = Type Cast(type=0, x=w787) -> (*(type *) &x=w785:i32)
            n250 = TCP Read(connection ID=w784, bytes to read=w785, error in (no error)=w783) -> (connection ID out=w779:refnum<k5>, data out=w782:string, error out=w778:errorcluster)  [unwired: 2 out]
            n251 = call "deleteEndString.vi"("chars to delete"=5, "string in"=w782) -> ("substring out"=w781:string)  [unwired: 9 out]
            n252 = call "searchElement.vi"("input"=w776, "name"=w781) -> ("output"=w789:cluster{"name":string, "type desc":i16[]})  [unwired: 9 out]
            n253 = Unbundle By Name(w789) -> ("name"=w788:string)
            n254 = invoke class="VI" method="Ctrl Val.Get (Deprecated)"(reference=w773, error in=w772, "Control Name"=w788) -> (reference out=w771:refnum<vi>, error out=w770:errorcluster, "Get Control Value"=w777:string)  [unwired: 2 in, 2 out]
            n255 = TCP Write(connection ID=w779, data in=w777, error in (no error)=w778) -> (connection ID out=w769:refnum<k5>, error out=w768:errorcluster)  [unwired: 2 out]
          }
          frame "getIntArray" {
            n256 = TCP Read(connection ID=w799, bytes to read=4, error in (no error)=w798) -> (connection ID out=w807:refnum<k5>, data out=w810:string, error out=w806:errorcluster)  [unwired: 2 out]
            n257 = Type Cast(type=0, x=w810) -> (*(type *) &x=w808:i32)
            n258 = TCP Read(connection ID=w807, bytes to read=w808, error in (no error)=w806) -> (connection ID out=w802:refnum<k5>, data out=w805:string, error out=w801:errorcluster)  [unwired: 2 out]
            n259 = call "deleteEndString.vi"("chars to delete"=5, "string in"=w805) -> ("substring out"=w804:string)  [unwired: 9 out]
            n260 = call "searchElement.vi"("input"=w793, "name"=w804) -> ("output"=w812:cluster{"name":string, "type desc":i16[]})  [unwired: 9 out]
            n261 = Unbundle By Name(w812) -> ("name"=w811:string)
            n262 = invoke class="VI" method="Ctrl Val.Get (Deprecated)"(reference=w796, error in=w797, "Control Name"=w811) -> (reference out=w794:refnum<vi>, error out=w795:errorcluster, "Get Control Value"=w800:string)  [unwired: 2 in, 2 out]
            n263 = TCP Write(connection ID=w802, data in=w800, error in (no error)=w801) -> (connection ID out=w792:refnum<k5>, error out=w791:errorcluster)  [unwired: 2 out]
          }
          frame "getDoubleArray" {
            n264 = TCP Read(connection ID=w821, bytes to read=4, error in (no error)=w822) -> (connection ID out=w830:refnum<k5>, data out=w833:string, error out=w829:errorcluster)  [unwired: 2 out]
            n265 = Type Cast(type=0, x=w833) -> (*(type *) &x=w831:i32)
            n266 = TCP Read(connection ID=w830, bytes to read=w831, error in (no error)=w829) -> (connection ID out=w825:refnum<k5>, data out=w828:string, error out=w824:errorcluster)  [unwired: 2 out]
            n267 = call "deleteEndString.vi"("chars to delete"=5, "string in"=w828) -> ("substring out"=w827:string)  [unwired: 9 out]
            n268 = call "searchElement.vi"("input"=w816, "name"=w827) -> ("output"=w835:cluster{"name":string, "type desc":i16[]})  [unwired: 9 out]
            n269 = Unbundle By Name(w835) -> ("name"=w834:string)
            n270 = invoke class="VI" method="Ctrl Val.Get (Deprecated)"(reference=w819, error in=w820, "Control Name"=w834) -> (reference out=w817:refnum<vi>, error out=w818:errorcluster, "Get Control Value"=w823:string)  [unwired: 2 in, 2 out]
            n271 = TCP Write(connection ID=w825, data in=w823, error in (no error)=w824) -> (connection ID out=w815:refnum<k5>, error out=w814:errorcluster)  [unwired: 2 out]
          }
          frame "getStringArray" {
            n272 = TCP Read(connection ID=w845, bytes to read=4, error in (no error)=w844) -> (connection ID out=w853:refnum<k5>, data out=w856:string, error out=w852:errorcluster)  [unwired: 2 out]
            n273 = Type Cast(type=0, x=w856) -> (*(type *) &x=w854:i32)
            n274 = TCP Read(connection ID=w853, bytes to read=w854, error in (no error)=w852) -> (connection ID out=w848:refnum<k5>, data out=w851:string, error out=w847:errorcluster)  [unwired: 2 out]
            n275 = call "deleteEndString.vi"("chars to delete"=5, "string in"=w851) -> ("substring out"=w850:string)  [unwired: 9 out]
            n276 = call "searchElement.vi"("input"=w839, "name"=w850) -> ("output"=w858:cluster{"name":string, "type desc":i16[]})  [unwired: 9 out]
            n277 = Unbundle By Name(w858) -> ("name"=w857:string)
            n278 = invoke class="VI" method="Ctrl Val.Get (Deprecated)"(reference=w842, error in=w843, "Control Name"=w857) -> (reference out=w840:refnum<vi>, error out=w841:errorcluster, "Get Control Value"=w846:string)  [unwired: 2 in, 2 out]
            n279 = TCP Write(connection ID=w848, data in=w846, error in (no error)=w847) -> (connection ID out=w838:refnum<k5>, error out=w837:errorcluster)  [unwired: 2 out]
          }
          frame "getFloatArray" {
            n280 = TCP Read(connection ID=w866, bytes to read=4, error in (no error)=w865) -> (connection ID out=w876:refnum<k5>, data out=w879:string, error out=w875:errorcluster)  [unwired: 2 out]
            n281 = Type Cast(type=0, x=w879) -> (*(type *) &x=w877:i32)
            n282 = TCP Read(connection ID=w876, bytes to read=w877, error in (no error)=w875) -> (connection ID out=w871:refnum<k5>, data out=w874:string, error out=w870:errorcluster)  [unwired: 2 out]
            n283 = call "deleteEndString.vi"("chars to delete"=5, "string in"=w874) -> ("substring out"=w873:string)  [unwired: 9 out]
            n284 = call "searchElement.vi"("input"=w864, "name"=w873) -> ("output"=w881:cluster{"name":string, "type desc":i16[]})  [unwired: 9 out]
            n285 = Unbundle By Name(w881) -> ("name"=w880:string)
            n286 = invoke class="VI" method="Ctrl Val.Get (Deprecated)"(reference=w867, error in=w868, "Control Name"=w880) -> (reference out=w863:refnum<vi>, error out=w862:errorcluster, "Get Control Value"=w869:string)  [unwired: 2 in, 2 out]
            n287 = TCP Write(connection ID=w871, data in=w869, error in (no error)=w870) -> (connection ID out=w861:refnum<k5>, error out=w860:errorcluster)  [unwired: 2 out]
          }
          frame "getBooleanArray2D" {
            n288 = TCP Read(connection ID=w890, bytes to read=4, error in (no error)=w891) -> (connection ID out=w899:refnum<k5>, data out=w902:string, error out=w898:errorcluster)  [unwired: 2 out]
            n289 = Type Cast(type=0, x=w902) -> (*(type *) &x=w900:i32)
            n290 = TCP Read(connection ID=w899, bytes to read=w900, error in (no error)=w898) -> (connection ID out=w894:refnum<k5>, data out=w897:string, error out=w893:errorcluster)  [unwired: 2 out]
            n291 = call "deleteEndString.vi"("chars to delete"=5, "string in"=w897) -> ("substring out"=w896:string)  [unwired: 9 out]
            n292 = call "searchElement.vi"("input"=w885, "name"=w896) -> ("output"=w904:cluster{"name":string, "type desc":i16[]})  [unwired: 9 out]
            n293 = Unbundle By Name(w904) -> ("name"=w903:string)
            n294 = invoke class="VI" method="Ctrl Val.Get (Deprecated)"(reference=w888, error in=w889, "Control Name"=w903) -> (reference out=w886:refnum<vi>, error out=w887:errorcluster, "Get Control Value"=w892:string)  [unwired: 2 in, 2 out]
            n295 = TCP Write(connection ID=w894, data in=w892, error in (no error)=w893) -> (connection ID out=w884:refnum<k5>, error out=w883:errorcluster)  [unwired: 2 out]
          }
          frame "getIntArray2D" {
            n296 = TCP Read(connection ID=w914, bytes to read=4, error in (no error)=w913) -> (connection ID out=w922:refnum<k5>, data out=w925:string, error out=w921:errorcluster)  [unwired: 2 out]
            n297 = Type Cast(type=0, x=w925) -> (*(type *) &x=w923:i32)
            n298 = TCP Read(connection ID=w922, bytes to read=w923, error in (no error)=w921) -> (connection ID out=w917:refnum<k5>, data out=w920:string, error out=w916:errorcluster)  [unwired: 2 out]
            n299 = call "deleteEndString.vi"("chars to delete"=5, "string in"=w920) -> ("substring out"=w919:string)  [unwired: 9 out]
            n300 = call "searchElement.vi"("input"=w908, "name"=w919) -> ("output"=w927:cluster{"name":string, "type desc":i16[]})  [unwired: 9 out]
            n301 = Unbundle By Name(w927) -> ("name"=w926:string)
            n302 = invoke class="VI" method="Ctrl Val.Get (Deprecated)"(reference=w911, error in=w912, "Control Name"=w926) -> (reference out=w909:refnum<vi>, error out=w910:errorcluster, "Get Control Value"=w915:string)  [unwired: 2 in, 2 out]
            n303 = TCP Write(connection ID=w917, data in=w915, error in (no error)=w916) -> (connection ID out=w907:refnum<k5>, error out=w906:errorcluster)  [unwired: 2 out]
          }
          frame "getDoubleArray2D" {
            n304 = TCP Read(connection ID=w936, bytes to read=4, error in (no error)=w937) -> (connection ID out=w945:refnum<k5>, data out=w948:string, error out=w944:errorcluster)  [unwired: 2 out]
            n305 = Type Cast(type=0, x=w948) -> (*(type *) &x=w946:i32)
            n306 = TCP Read(connection ID=w945, bytes to read=w946, error in (no error)=w944) -> (connection ID out=w940:refnum<k5>, data out=w943:string, error out=w939:errorcluster)  [unwired: 2 out]
            n307 = call "deleteEndString.vi"("chars to delete"=5, "string in"=w943) -> ("substring out"=w942:string)  [unwired: 9 out]
            n308 = call "searchElement.vi"("input"=w931, "name"=w942) -> ("output"=w950:cluster{"name":string, "type desc":i16[]})  [unwired: 9 out]
            n309 = Unbundle By Name(w950) -> ("name"=w949:string)
            n310 = invoke class="VI" method="Ctrl Val.Get (Deprecated)"(reference=w934, error in=w935, "Control Name"=w949) -> (reference out=w932:refnum<vi>, error out=w933:errorcluster, "Get Control Value"=w938:string)  [unwired: 2 in, 2 out]
            n311 = TCP Write(connection ID=w940, data in=w938, error in (no error)=w939) -> (connection ID out=w930:refnum<k5>, error out=w929:errorcluster)  [unwired: 2 out]
          }
          frame "getStringArray2D" {
            n312 = TCP Read(connection ID=w959, bytes to read=4, error in (no error)=w960) -> (connection ID out=w968:refnum<k5>, data out=w971:string, error out=w967:errorcluster)  [unwired: 2 out]
            n313 = Type Cast(type=0, x=w971) -> (*(type *) &x=w969:i32)
            n314 = TCP Read(connection ID=w968, bytes to read=w969, error in (no error)=w967) -> (connection ID out=w963:refnum<k5>, data out=w966:string, error out=w962:errorcluster)  [unwired: 2 out]
            n315 = call "deleteEndString.vi"("chars to delete"=5, "string in"=w966) -> ("substring out"=w965:string)  [unwired: 9 out]
            n316 = call "searchElement.vi"("input"=w954, "name"=w965) -> ("output"=w973:cluster{"name":string, "type desc":i16[]})  [unwired: 9 out]
            n317 = Unbundle By Name(w973) -> ("name"=w972:string)
            n318 = invoke class="VI" method="Ctrl Val.Get (Deprecated)"(reference=w957, error in=w958, "Control Name"=w972) -> (reference out=w955:refnum<vi>, error out=w956:errorcluster, "Get Control Value"=w961:string)  [unwired: 2 in, 2 out]
            n319 = TCP Write(connection ID=w963, data in=w961, error in (no error)=w962) -> (connection ID out=w953:refnum<k5>, error out=w952:errorcluster)  [unwired: 2 out]
          }
          frame "getFloatArray2D" {
            n320 = TCP Read(connection ID=w983, bytes to read=4, error in (no error)=w982) -> (connection ID out=w991:refnum<k5>, data out=w994:string, error out=w990:errorcluster)  [unwired: 2 out]
            n321 = Type Cast(type=0, x=w994) -> (*(type *) &x=w992:i32)
            n322 = TCP Read(connection ID=w991, bytes to read=w992, error in (no error)=w990) -> (connection ID out=w986:refnum<k5>, data out=w989:string, error out=w985:errorcluster)  [unwired: 2 out]
            n323 = call "deleteEndString.vi"("chars to delete"=5, "string in"=w989) -> ("substring out"=w988:string)  [unwired: 9 out]
            n324 = call "searchElement.vi"("input"=w981, "name"=w988) -> ("output"=w996:cluster{"name":string, "type desc":i16[]})  [unwired: 9 out]
            n325 = Unbundle By Name(w996) -> ("name"=w995:string)
            n326 = invoke class="VI" method="Ctrl Val.Get (Deprecated)"(reference=w978, error in=w977, "Control Name"=w995) -> (reference out=w979:refnum<vi>, error out=w980:errorcluster, "Get Control Value"=w984:string)  [unwired: 2 in, 2 out]
            n327 = TCP Write(connection ID=w986, data in=w984, error in (no error)=w985) -> (connection ID out=w976:refnum<k5>, error out=w975:errorcluster)  [unwired: 2 out]
          }
        }
        n328 = property class="VI"(reference=w49, error in=w48) -> (reference out=w40:refnum<vi>, error out=w41:errorcluster, "Exec.State"=w45:T1)
        "error out 2" <- w41
        n329 = Unbundle By Name(w53) -> ("status"=w50:bool)
        n330 = call "stopVILV2G.vi"("Mode"=enum16{"Init", "Get", "Set"}."Get") -> ("Stop OUT"=w51:bool)  [unwired: 1 in, 9 out]
        n331 = Unbundle By Name(w41) -> ("status"=w46:bool)
        n332 = Equal?(x=w45, y=T1."Idle" ("x")) -> (x = y?=w47:bool)
        n333 = Compound Arithmetic op=OR(w46, w47, w50, w51) -> (w42:bool)
      }
    }
  }
  "connection ID out" <- w8
  "error TCP out" <- w7
  n334 = case shown="True" w2 {
    tunnel: [w999 w1022] -> w6
    tunnel: [w998 w1021] -> w5
    tunnel: w3 -> [w999 w1012]
    tunnel: w4 -> [w998 w1009]
    tunnel: "input Controls" -> [_ w1000]
    frame False {
    }
    frame True {
      # "It detects if the VI has a boolean variable named \"stop\". If this is so, then it will try to stop the VI sending a TRUE value to this variable.\nNotice that client must use a TRUE value to the stop boolean variable when he wants stop his VI application."
      # "if the VI of the client still is running because it hasn't a \"stop\" labelled variable (boolean), then the VI will be aborted.\nNotice that it isn't a good practice when you use hardware in the loop. In this case, you need to use a variable named \"stop\" to finalize the VI and put the actuator to zero of a clean way."
      # "Reinit All values in the VI before of closing the Reference."
      n335 = Array Size(array=w1000) -> (size(s)=w1020:i32)
      n336 = property class="VI"(reference=w1012, error in=w1009) -> (reference out=w1011:refnum<vi>, error out=w1010:errorcluster, "Exec.State"=w1004:T1)
      n337 = Greater Than 0?(x=w1020) -> (x > 0?=w1008:bool)
      n338 = Equal?(x=w1004, y=T1."Running") -> (x = y?=w1005:bool)
      n339 = Equal?(x=w1004, y=T1."Run top level") -> (x = y?=w1002:bool)
      n340 = Or(x=w1005, y=w1002) -> (x .or. y?=w1001:bool)
      n341 = And(x=w1008, y=w1001) -> (x .and. y?=w1007:bool)
      n342 = case shown="True" w1007 {
        tunnel: w1000 -> [_ w1040]
        tunnel: w1020 -> [_ w1039]
        tunnel: w1011 -> [w1034 w1038]
        tunnel: w1010 -> [w1033 w1037]
        tunnel: [w1034 w1036] -> w1018
        tunnel: [w1033 w1035] -> w1017
        frame False {
        }
        frame True {
          n343 = while {
            tunnel: w1040 -> [w1049] mode=indexing
            tunnel: w1039 -> [w1052]
            tunnel: w1038 -> [w1047]
            tunnel: w1037 -> [w1046]
            tunnel: [w1042] -> w1036
            tunnel: [w1041] -> w1035
            i -> [w1053]
            stop <- w1054 stop-if-true
            w1043 = "stop" ("y")
            n344 = Unbundle By Name(w1049) -> ("name"=w1044:string, "type desc"=w1045:i16[])
            n345 = Equal?(x=w1043, y=w1044) -> (x = y?=w1048:bool)
            n346 = case shown="True" w1048 {
              tunnel: w1047 -> [w1056 w1065]
              tunnel: w1046 -> [w1055 w1064]
              tunnel: w1045 -> [_ w1061]
              tunnel: w1043 -> [_ w1060]
              tunnel: [w1056 w1059] -> w1042
              tunnel: [w1055 w1058] -> w1041
              frame False {
              }
              frame True {
                n347 = Variant To Flattened String(Variant=TRUE) -> (data string=w1062:string)  [unwired: 1 out]
                n348 = invoke class="VI" method="Ctrl Val.Set (Deprecated)"(reference=w1065, error in=w1064, "Control Name"=w1060, "Type Descriptor"=w1061, "Flattened Data"=w1062) -> (reference out=w1059:refnum<vi>, error out=w1058:errorcluster)  [unwired: 1 in, 4 out]
                n349 = Wait (ms)(milliseconds to wait=u32 100 ("millisecond multiple")) -> ()  [unwired: 1 out]
              }
            }
            n350 = Decrement(x=w1052) -> (x-1=w1051:i32)
            n351 = Equal?(x=w1051, y=w1053) -> (x = y?=w1050:bool)
            n352 = Or(x=w1048, y=w1050) -> (x .or. y?=w1054:bool)
          }
        }
      }
      n353 = property class="VI"(reference=w1018, error in=w1017) -> (reference out=w1016:refnum<vi>, error out=w1015:errorcluster, "Exec.State"=w1019:T1)
      n354 = case shown="\"Running\"" w1019 {
        tunnel: w1016 -> [w1024 w1026 w1028 w1032]
        tunnel: w1015 -> [w1023 w1025 w1027 w1031]
        tunnel: [w1024 w1026 w1028 w1030] -> w1014
        tunnel: [w1023 w1025 w1027 w1029] -> w1013
        frame "Bad", Default {
        }
        frame "Idle" {
        }
        frame "Run top level" {
        }
        frame "Running" {
          n355 = invoke class="VI" method="Abort VI"(reference=w1032, error in=w1031) -> (reference out=w1030:refnum<vi>, error out=w1029:errorcluster)  [unwired: 1 in, 1 out]
        }
      }
      n356 = invoke class="VI" method="Default Vals.Reinit All"(reference=w1014, error in=w1013) -> (reference out=w1022:refnum<vi>, error out=w1021:errorcluster)  [unwired: 1 in, 1 out]
    }
  }
  "vi reference" <- w6
  "error out" <- w5
